vi "Get Turbo Valve Value.vi"(8 "error in (no error)":errorcluster, 11 "ILC TV Open Loop Actuator Cylinder in":refnum<class "ILC TV Open Loop Actuator Cylinder.lvclass">) -> (0 "error out":errorcluster, 2 "Value":dbl format="%.2f", 3 "ILC TV Open Loop Actuator Cylinder out":refnum<class "ILC TV Open Loop Actuator Cylinder.lvclass">)   [LabVIEW 2015, in "ILC TV Open Loop Actuator Cylinder.lvclass"]
uses:
  ILC TV Open Loop Actuator Cylinder.lvclass
  ILC Actuator Cylinder/ILC Actuator Cylinder.lvclass/ILC Actuator Cylinder.ctl
  ILC Actuator Cylinder/ILC Actuator Cylinder.lvclass
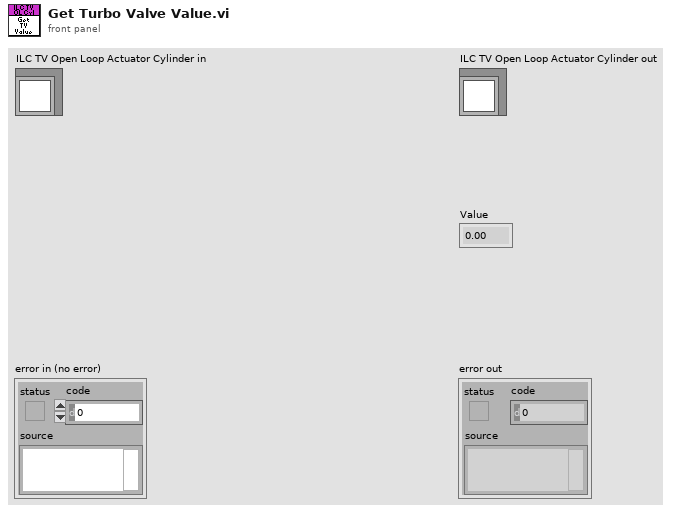
[diagram p1: front panel]
types:
  T1 = typedef "FAMT Typedefs.lvlib/Turbo Valve Settings.ctl" = cluster{"ROT Bias":u8, "Minimum Voltage":dbl, "Maximum Voltage":dbl, "Off Value":dbl}
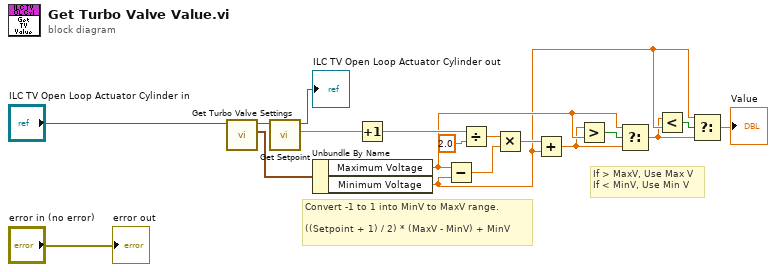
[diagram p0: block diagram]
diagram:
  # "If > MaxV, Use Max V\nIf < MinV, Use Min V"
  # "Convert -1 to 1 into MinV to MaxV range.\n\n((Setpoint + 1) / 2) * (MaxV - MinV) + MinV"
  n1 = call "Get Turbo Valve Settings.vi"("ILC Actuator Cylinder in"="ILC TV Open Loop Actuator Cylinder in") -> ("Turbo Valve Settings"=w14:T1, "ILC Actuator Cylinder out"=w15:refnum<class "ILC TV Open Loop Actuator Cylinder.lvclass">)  [unwired: 9 in]
  n2 = call-dynamic "Get Setpoint.vi"("ILC Actuator Cylinder in"=w15) -> ("Setpoint"=w13:dbl, "ILC Actuator Cylinder out"=→"ILC TV Open Loop Actuator Cylinder out":refnum<class "ILC TV Open Loop Actuator Cylinder.lvclass">)  [unwired: 9 in]
  n3 = Unbundle By Name(w14) -> ("Maximum Voltage"=w6:dbl, "Minimum Voltage"=w3:dbl)
  n4 = Increment(x=w13) -> (x+1=w12:dbl)
  n5 = Subtract(x=w6, y=w3) -> (x-y=w9:dbl)
  n6 = Divide(x=w12, y=2.0) -> (x/y=w10:dbl)
  n7 = Multiply(x=w10, y=w9) -> (x*y=w8:dbl)
  n8 = Add(x=w8, y=w3) -> (x+y=w5:dbl)
  n9 = Greater?(x=w5, y=w6) -> (0:w7:bool)
  n10 = Select(t=w6, s=w7, f=w5) -> (s? t:f=w2:dbl)
  n11 = Less?(x=w2, y=w3) -> (x < y?=w4:bool)
  n12 = Select(t=w3, s=w4, f=w2) -> (s? t:f=→"Value":dbl)
  "error out" <- "error in (no error)"
